vi "HackRF_Read.vi"   [LabVIEW 2010]
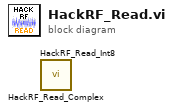
[diagram p0: block diagram]
diagram:
  n1 = call "HackRF_Read_Complex.vi"() -> ()  [unwired: 9 in, 3 out]
  n2 = call "HackRF_Read_Int8.vi"() -> ()  [unwired: 8 in, 4 out]
